vi "Insert value by reference.vi"(8 "error in (no error)":errorcluster, 10 "Control in":refnum<vi>, 11 "Variant value IN":variant) -> (0 "error out":errorcluster)   [LabVIEW 2020]
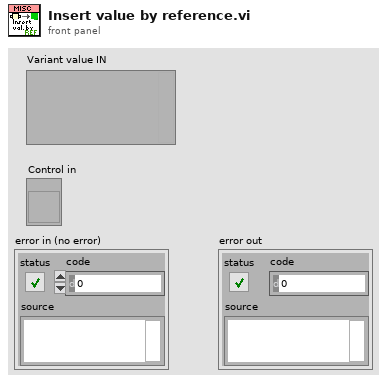
[diagram p1: front panel]
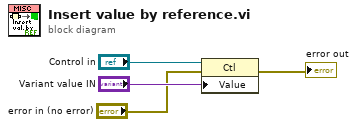
[diagram p0: block diagram]
diagram:
  n1 = property class="Ctl"(reference="Control in", error in="error in (no error)", "Value"="Variant value IN") -> (error out=→"error out":errorcluster)  [unwired: 1 out]
